vi "Element by Name.vi"(8 "error in (no error)":errorcluster, 10 "Full Name":string, 11 "Config Manager in":refnum<class "Config Manager.lvclass">) -> (0 "error out":errorcluster, 2 "Config Element":refnum<class "Config Element.lvclass">, 3 "Config Manager out":refnum<class "Config Manager.lvclass">)   [LabVIEW 2020, in "CDM-Config.lvlib" / "Config Manager.lvclass"]
uses:
  Config Manager.lvclass
  Config Element/Config Element.lvclass
  Config Manager.lvclass/Config Manager.ctl
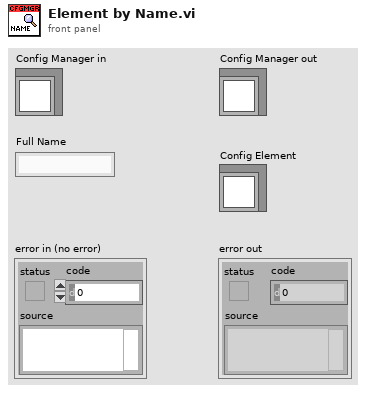
[diagram p1: front panel]
types:
  T1 = typedef "CDM-Config.lvlib/Config Manager.lvclass/Ref Data.ctl" = cluster{"Elements":refnum<class "Config Element.lvclass">[], "Name Separator":string, "Hierarchy Map":map{string[], i32}, "Meta Name Map":map{string, i32[]}}
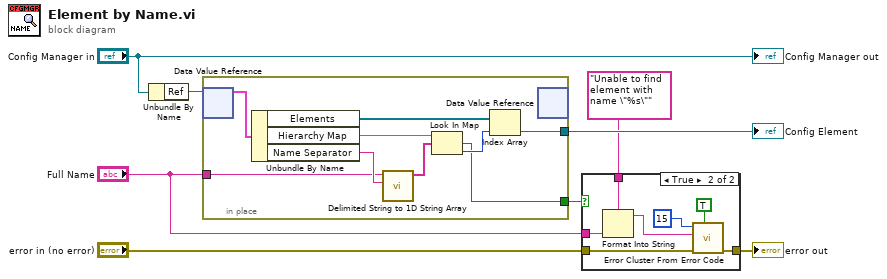
[diagram p0: block diagram]
diagram:
  n1 = Unbundle By Name("Config Manager in") -> ("Ref"=w7:refnum<data-value>)
  n2 = in-place {
    in-place-border: "Full Name" -> [w10]
    in-place-border: [w13] -> w6
    in-place-border: [w12] -> w4
    n3 = in-place-dvr #1(w7) -> (w17:T1)  [unwired: 1 out]
    n4 = Unbundle By Name(w17) -> ("Elements"=w15:refnum<class "Config Element.lvclass">[], "Hierarchy Map"=w16:map{string[], i32}, "Name Separator"=w11:string)
    n5 = call <vilib>:"Delimited String to 1D String Array.vi"("delimiter"=w11, "delimited string"=w10) -> ("string array"=w9:string[])  [unwired: 9 in]
    n6 = Look In Map(map=w16, key=w9) -> (key not found?=w12:bool, value=w14:i32)  [unwired: 1 in]
    n7 = Index Array(array=w15, index=w14) -> (element=w13:refnum<class "Config Element.lvclass">)
    n8 = in-place-dvr #1() -> ()  [unwired: 1 in, 2 out]
  }
  "Config Element" <- w6
  n9 = case shown="True" w4 {
    tunnel: "error in (no error)" -> [w18 w23]
    tunnel: [w18 w22] -> w3
    tunnel: "Full Name" -> [_ w25]
    tunnel: "Unable to find element with name \"%s\"" -> [_ w24]
    frame False {
    }
    frame True {
      n10 = Format Into String(format string=w24, w25) -> (resulting string=w19:string)  [unwired: 2 in, 1 out]
      n11 = call <vilib>:"Error Cluster From Error Code.vi"("show call chain? (False)"=TRUE, "error in (no error)"=w23, "error message (\"\")"=w19, "error code (0)"=15) -> ("error out"=w22:errorcluster)  [unwired: 5 in]
    }
  }
  "error out" <- w3
  "Config Manager out" <- "Config Manager in"
